vi "Write And Read Tag.vi"() -> ()   [LabVIEW 2019]
doc: "Demonstrates how to write and read data of Logix tags in a PLC. The PLC must support Messaging class communications."
uses:
  <vilib>/ethernetip/ethernetip.llb/EthernetIP Tag Read SINT.vi
  <vilib>/ethernetip/ethernetip.llb/EthernetIP Tag Read BOOL.vi
  <vilib>/ethernetip/ethernetip.llb/EthernetIP Tag Write SINT.vi
  <vilib>/ethernetip/ethernetip.llb/EthernetIP Tag Write BOOL.vi
  <vilib>/ethernetip/ethernetip.lvlib
panel:
  in  "BOOL data":bool[](array[boolean])
  out "SINT data":i8[](array[numeric])
  in  "SINT data":i8[](array[numeric])
  out "BOOL data":bool[](array[boolean])
  in  "stop reading":bool
  in  "reading rate [ms]":u32=500
  out "reading?":bool
  in  "number of SINT":u32=1
  in  "number of BOOL":u32=1
  in  "SINT tag":string="DataArray_SINT"
  in  "BOOL tag":string="DataArray_BOOL"
  in  "BOOL tag":string="DataArray_BOOL"
  in  "stop writing":bool
  out "writing?":bool
  in  "SINT tag":string="DataArray_SINT"
  in  "writing rate [ms]":u32=500
  in  "network path":string="*.*.*.*,*,*"
  in  "timeout [ms]":i32=1000
  # "Overview: Demonstrates how to write and read data of Logix tags in a PLC. The PLC must support Messaging class communications.\nRequirements: LabVIEW Base Development System, NI-Industrial Communications for Ethernet/IP, RSLogix 5000 Device\nInstructions:\n1. Create tags in a PLC device.\n2. Configure network path, timeout, writing rate, and reading rate.\n3. Set Write Data for writing data to Logix tags.\n4. Set corresponding tags in Read Data.\n5. Run this VI. This VI returns the tag values that you write.\n6. Click both Stop Writing and Stop Reading to stop this VI."
  # "Configuration"
  # "Write Data"
  # "Read Data"
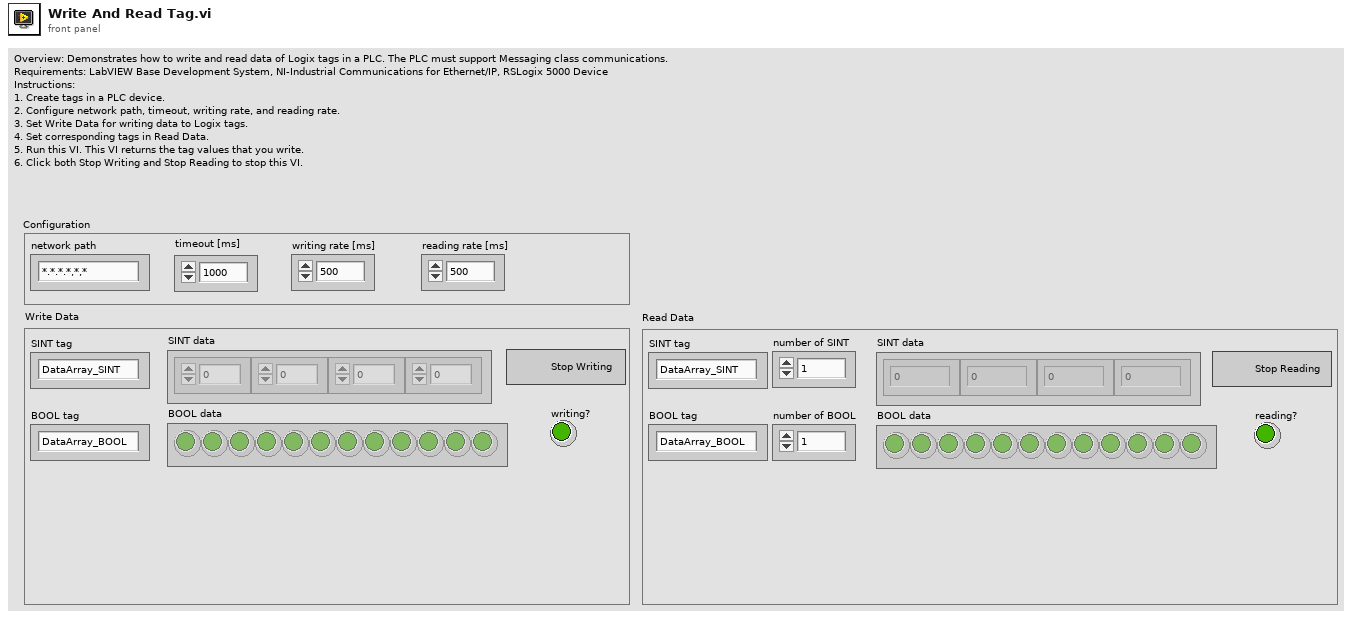
[diagram p1: front panel]
types:
  T1 = typedef "ethernetip.lvlib/ethernetip.ctl" = refnum<k21>
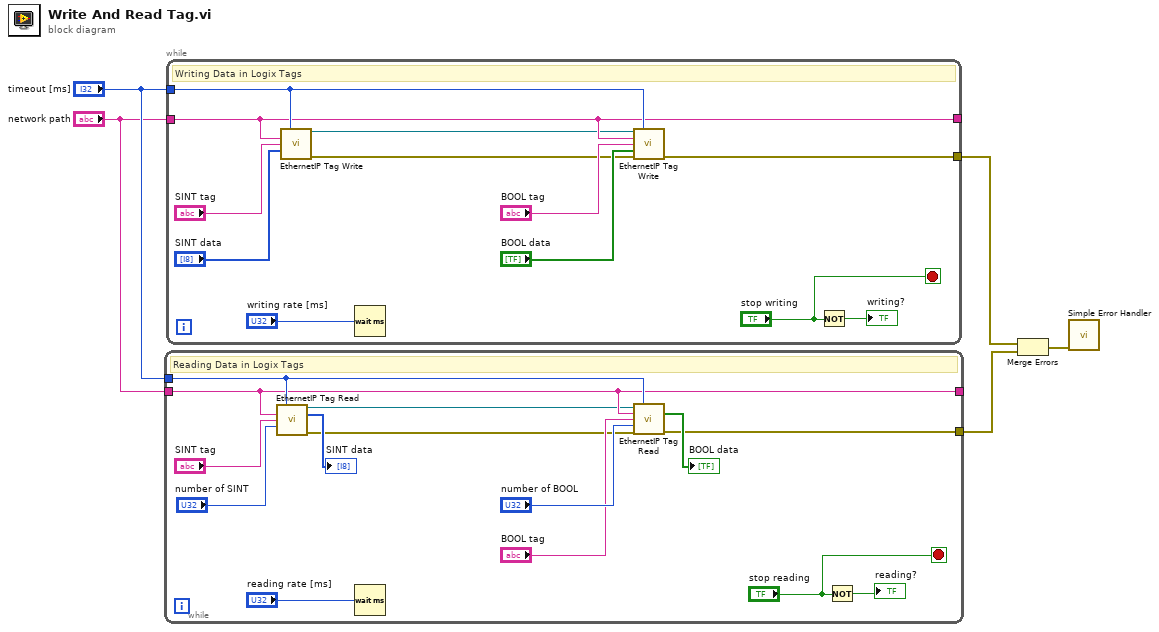
[diagram p0: block diagram]
diagram:
  n1 = while {
    tunnel: "timeout [ms]" -> [w11]
    tunnel: "network path" -> [w10]
    tunnel: [w8] -> w1
    tunnel: [w10] -> _
    stop <- "stop reading" stop-if-true
    # "Reading Data in Logix Tags"
    n2 = call-poly <vilib>:"EthernetIP Tag Read.vi"("Timeout (ms)"=w11, "Network Path"=w10, "Tag Name"="SINT tag", "Number of Elements"="number of SINT") -> ("Session out"=w7:T1, "Data"=→"SINT data":i8[], "error out"=w6:errorcluster)  [unwired: 2 in, 7 out]
    n3 = Wait (ms)(milliseconds to wait="reading rate [ms]") -> ()  [unwired: 1 out]
    n4 = call-poly <vilib>:"EthernetIP Tag Read.vi"("Session in"=w7, "Timeout (ms)"=w11, "Network Path"=w10, "Tag Name"="BOOL tag", "Number of Elements"="number of BOOL", "error in"=w6) -> ("Data"=→"BOOL data":bool[], "error out"=w8:errorcluster)  [unwired: 8 out]
    n5 = Not(x="stop reading") -> (.not. x?=→"reading?":bool)
  }
  n6 = while {
    tunnel: "network path" -> [w24]
    tunnel: "timeout [ms]" -> [w25]
    tunnel: [w20] -> w2
    tunnel: [w24] -> _
    stop <- "stop writing" stop-if-true
    # "Writing Data in Logix Tags"
    n7 = call-poly <vilib>:"EthernetIP Tag Write.vi"("Timeout (ms)"=w25, "Network Path"=w24, "Tag Name"="SINT tag", "Data"="SINT data") -> ("Session out"=w22:T1, "error out"=w21:errorcluster)  [unwired: 2 in, 8 out]
    n8 = Wait (ms)(milliseconds to wait="writing rate [ms]") -> ()  [unwired: 1 out]
    n9 = call-poly <vilib>:"EthernetIP Tag Write.vi"("Session in"=w22, "Timeout (ms)"=w25, "Network Path"=w24, "Tag Name"="BOOL tag", "Data"="BOOL data", "error in"=w21) -> ("error out"=w20:errorcluster)  [unwired: 9 out]
    n10 = Not(x="stop writing") -> (.not. x?=→"writing?":bool)
  }
  n11 = Merge Errors(w2, w1) -> (w5:errorcluster)
  n12 = call <vilib>:"Simple Error Handler.vi"("error in (no error)"=w5) -> ()  [unwired: 1 in, 8 out]
